vi "FGV_PROXY_DIAGNOSTICS_message_history_display.vi"(4 "front_panel_reference":refnum<vi>, 6 "SQL_listbox_reference":refnum<vi>, 7 "options":T2, 8 "error_in":errorcluster, 9 "station":T1, 11 "input":variant) -> (0 "error_out":errorcluster)   [LabVIEW 2020]
uses:
  FGV_PROXY_DIAGNOSTICS_message_history_display.ctl
  STATION/station.ctl
  DIAGNOSTICS_message_history_buffer/PROXY_DIAGNOSTICS_message_history_buffer_all_info.ctl
  _misc/DIAGNOSTICS_message_type.ctl
  _misc/AULocalize/SubVIs/Get Localized Phrase Compact Interface 1D.vi
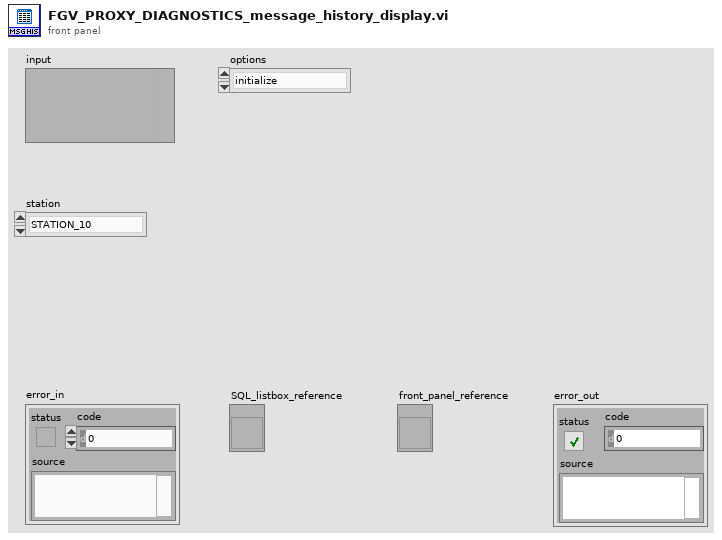
[diagram p1: front panel]
types:
  T1 = typedef "station.ctl" = enum16{"STATION_10", "STATION_20", "STATION_30", "STATION_40", "STATION_50", "STATION_60", "STATION_70", "STATION_80", "STATION_90", "STATION_100", "STATION_110", "STATION_120", "STATION_165", "MAIN"}
  T2 = typedef "FGV_PROXY_DIAGNOSTICS_message_history_display.ctl" = enum16{"initialize", "display_messages"}
  T3 = typedef "PROXY_DIAGNOSTICS_message_history_buffer_all_info.ctl" = cluster{"timestamp":timestamp, "station":T1, "message_type":T4, "message":string, "record":string[]}
  T4 = typedef "DIAGNOSTICS_message_type.ctl" = enum16{"TCP", "SQL"}
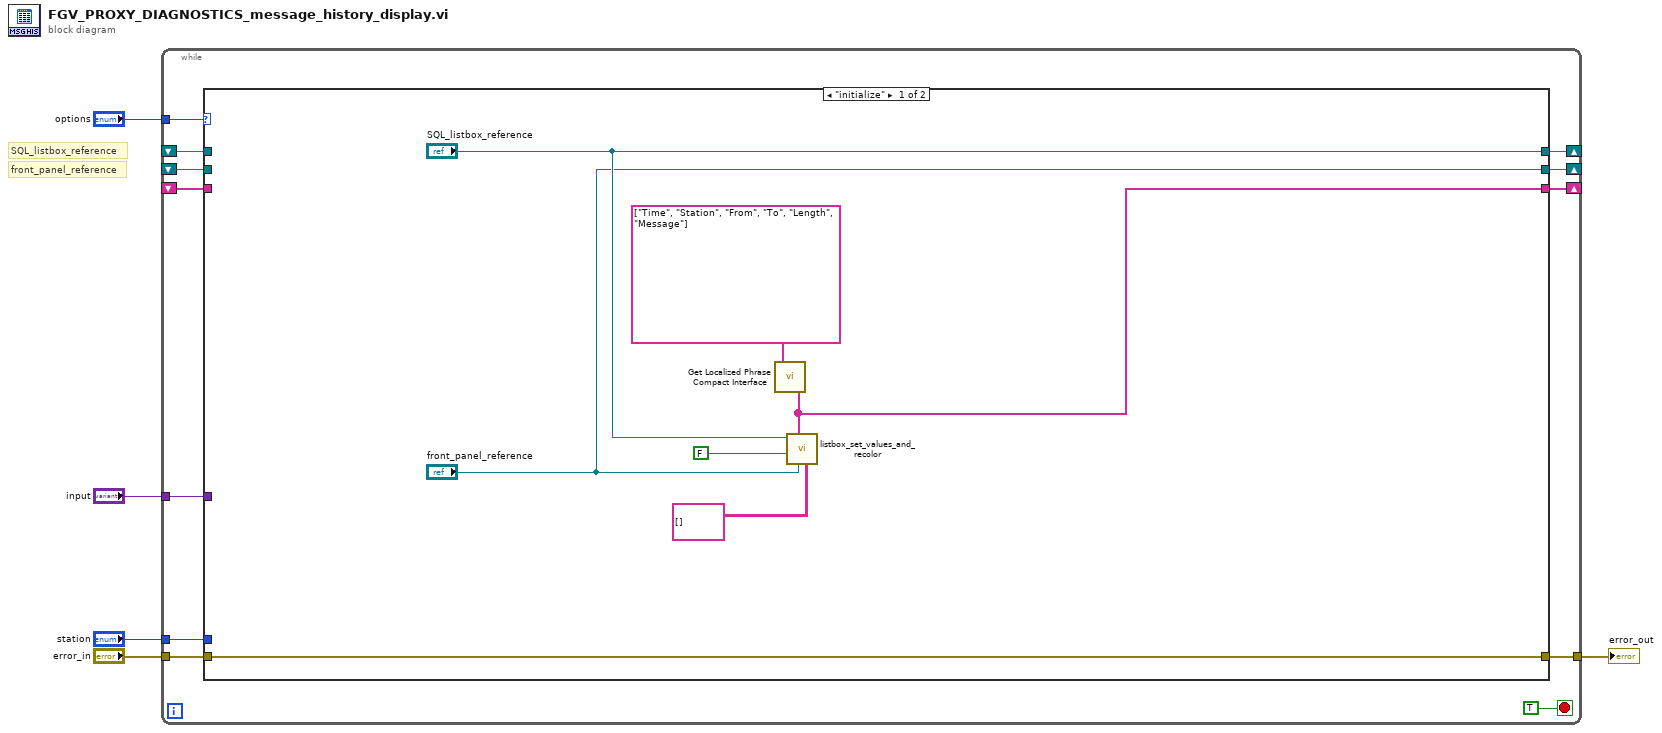
[diagram p0: block diagram]
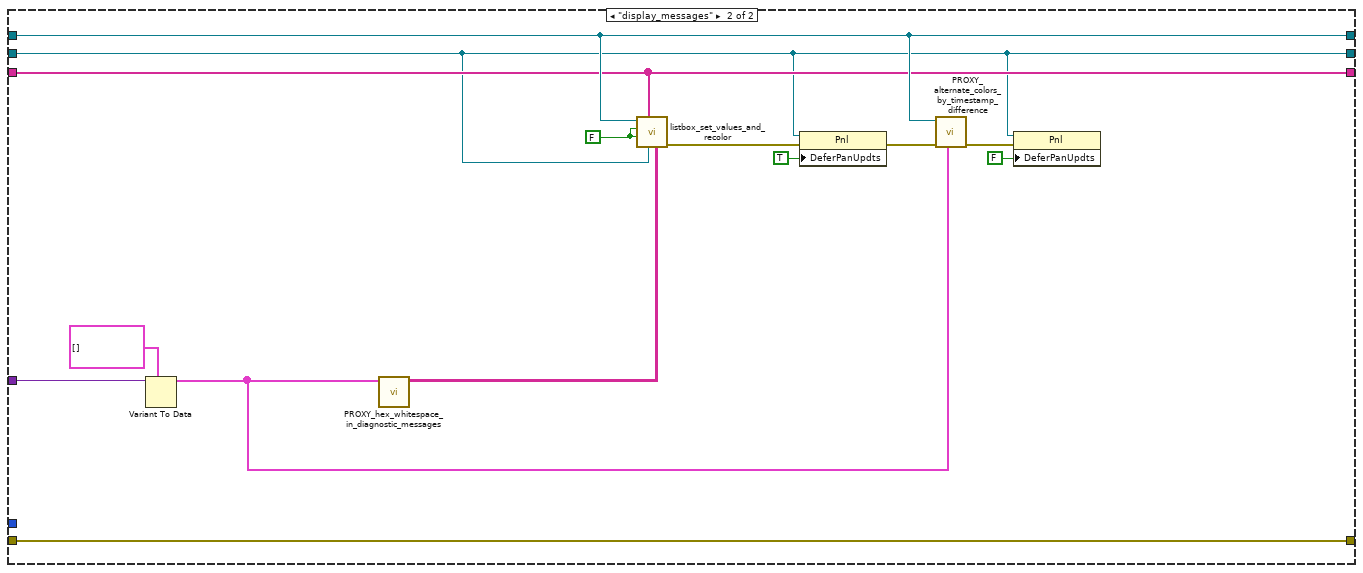
[diagram p2: hidden frame]
diagram:
  # "front_panel_reference"
  # "SQL_listbox_reference"
  n1 = while {
    tunnel: "options" -> [w16]
    tunnel: [w15] -> w5
    tunnel: "error_in" -> [w14]
    shift-right: [w13] -> _
    shift-left: _ -> [w12]
    tunnel: "input" -> [w11]
    shift-right: [w10] -> _
    shift-left: _ -> [w9]
    tunnel: "station" -> [w8]
    shift-right: [w7] -> _
    shift-left: _ -> [w6]
    stop <- TRUE stop-if-true
    n2 = case shown="\"initialize\"" w16 {
      tunnel: [w24 w38] -> w15
      tunnel: w14 -> [w24 w38]
      tunnel: ["SQL_listbox_reference" w32] -> w13
      tunnel: w12 -> [_ w32]
      tunnel: w11 -> [_ w37]
      tunnel: ["front_panel_reference" w27] -> w10
      tunnel: w9 -> [_ w27]
      tunnel: w8 -> [_ _]
      tunnel: [w18 w29] -> w7
      tunnel: w6 -> [_ w29]
      frame "initialize" {
        n3 = call-poly "Get Localized Phrase Compact Interface.vi"("Key"=string[] ["Time", "Station", "From", "To", "Length", "Message"] ("column_names")) -> ("Translated Phrase"=w18:string[])
        n4 = call "listbox_set_values_and_recolor.vi"("item_names"=string[][] [], "front_panel_reference"="front_panel_reference", "column_names"=w18, "Autosize? (T)"=FALSE, "multicolumn_listbox_reference_in"="SQL_listbox_reference") -> ()  [unwired: 5 in, 2 out]
      }
      frame "display_messages" {
        w31 = FALSE ("Autosize? (T)")
        n5 = Variant To Data(type=T3[] [] ("message_history"), Variant=w37) -> (data=w33:T3[])  [unwired: 1 in, 1 out]
        n6 = call "PROXY_hex_whitespace_in_diagnostic_messages.vi"("message_history"=w33) -> ("hexed_records"=w30:string[][])  [unwired: 10 in]
        n7 = call "listbox_set_values_and_recolor.vi"("item_names"=w30, "front_panel_reference"=w27, "column_names"=w29, "Autosize? (T)"=w31, "Recolor? (T)"=w31, "multicolumn_listbox_reference_in"=w32) -> ("error_out"=w26:errorcluster)  [unwired: 4 in, 1 out]
        n8 = property on="Property Node" class="Pnl"(reference=w27, error in=w26, "DeferPanUpdts"=TRUE ("Defer Panel Updates")) -> (error out=w25:errorcluster)  [unwired: 1 out]
        n9 = call "PROXY_alternate_colors_by_timestamp_difference.vi"("message_history_buffer"=w33, "error_in"=w25, "listbox_ref"=w32) -> ("error_out"=w34:errorcluster)  [unwired: 8 in]
        n10 = property on="Property Node" class="Pnl"(reference=w27, error in=w34, "DeferPanUpdts"=FALSE ("Defer Panel Updates")) -> ()  [unwired: 2 out]
      }
    }
  }
  "error_out" <- w5
